vi "Teleop.vi"(10 "Match Info":T1={"Autonomous Elapsed Seconds"=0.0, "TeleOp Elapsed Seconds"=0.0, "Disabled Elapsed Seconds"=0.0, "Visited Autonomous"=FALSE, "Visited TeleOp"=FALSE, "Visited Disabled"=FALSE, "Autonomous Settings"={"Autonomous Style"=enum."Independent", "VI Refnum"=refnum}}, 11 "Call Context":T2) -> ()   [LabVIEW 2013]
doc: "This VI is called for each TeleOp packet received from the DS where the robot is not disabled. It is often used to read from the joysticks and update I/O or to update setpoints for timed control loops. It should complete and return within 20 milliseconds or it may miss DS packets."
uses:
  <vilib>/Rock Robotics/WPI/DriverStation/WPI_DriverStationDerivedRobotMode.ctl
  <vilib>/Rock Robotics/WPI/DriverStation/WPI_DriverStationMatch Info.ctl
  <vilib>/Rock Robotics/WPI/Solenoid/WPI_SolenoidValue.ctl
  Robot Global Data.vi
  <vilib>/Rock Robotics/WPI/Solenoid/WPI_SolenoidSetEnum.vi
  <vilib>/Rock Robotics/WPI/Joystick/WPI_JoystickGetSetRefNum.vi
  <vilib>/Rock Robotics/WPI/Solenoid/WPI_SolenoidGetEnum.vi
  <vilib>/Rock Robotics/WPI/RobotDrive/WPI_RobotDriveGetSetRefNum.vi
  <vilib>/Rock Robotics/WPI/RobotDrive/WPI_RobotDriveMecanumDrive_Cartesian.vi
  <vilib>/Rock Robotics/WPI/RobotDrive/WPI_RobotDriveArcadeDrive_Standard(NoSaturation).vi
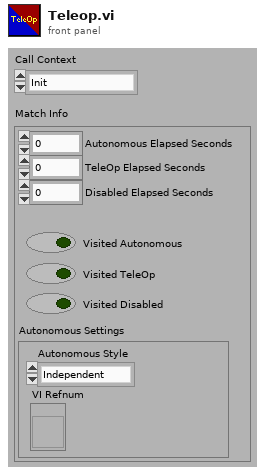
[diagram p1: front panel]
types:
  T1 = typedef "WPI_DriverStationMatch Info.ctl" = cluster{"Autonomous Elapsed Seconds":dbl, "TeleOp Elapsed Seconds":dbl, "Disabled Elapsed Seconds":dbl, "Visited Autonomous":bool, "Visited TeleOp":bool, "Visited Disabled":bool, "Autonomous Settings":cluster{"Autonomous Style":enum16{"Iterative", "Independent"}, "VI Refnum":refnum<vi>}}
  T2 = typedef "WPI_DriverStationDerivedRobotMode.ctl" = enum16{"Init", "Execute", "Stop"}
  T3 = cluster{"axis 1 (x)":dbl, "axis 2 (y)":dbl, "axis 3 (throttle)":dbl, "axis 4":dbl, "axis 5":dbl, "axis 6":dbl}
  T4 = typedef "WPI_JoystickDevRef.ctl" = cluster{"Device":T5}
  T5 = typedef "WPI_JoystickDeviceEnum.ctl" = enum16{"USB 1", "USB 2", "USB 3", "USB 4", "Kinect 1", "Kinect 2"}
  T6 = typedef "WPI_JoystickButtonState.ctl" = cluster{"Button 1":bool, "Button 2":bool, "Button 3":bool, "Button 4":bool, "Button 5":bool, "Button 6":bool, "Button 7":bool, "Button 8":bool, "Button 9":bool, "Button 10":bool, "Button 11":bool, "Button 12":bool}
  T7 = typedef "WPI_RobotDriveDevRef.ctl" = cluster{"DevStatus":errorcluster, "Motors[]":T8[], "Square Inputs":bool, "Max Output":dbl, "Isochronous":bool}
  T8 = typedef "WPI_MotorControlDeviceRef.ctl" = cluster{"DeviceStatus":errorcluster, "Type":enum16{"PWM", "CAN"}, "PWM":cluster{"Digital Module":T9, "PWM Channel":T10, "DeadBand":T11}, "CAN":cluster{"Device Number":u8, "Control Mode":T12, "Semaphore":T13, "Max Vout":dbl}, "Invert":bool, "TransformRef":T14, "InvTransformRef":T14}
  T9 = typedef "FPGA_TypedefDigitalModule.ctl" = enum16{"Digital Module 1", "Digital Module 2"}
  T10 = typedef "FPGA_DIOPWMChannel.ctl" = enum8{"PWM 1", "PWM 2", "PWM 3", "PWM 4", "PWM 5", "PWM 6", "PWM 7", "PWM 8", "PWM 9", "PWM 10", "Invalid"}
  T11 = typedef "WPI_PWMDeadband.ctl" = cluster{"Name":string, "maxPositivePwm":i32, "minPositivePwm":i32, "centerPwm":i32, "maxNegativePwm":i32, "minNegativePwm":i32, "angularRange":u16}
  T12 = typedef "WPI_CANJaguar_ControlMode.ctl" = enum8{"Percent VBus", "Current", "Speed", "Position", "Voltage"}
  T13 = typedef "Semaphore RefNum" = refnum<k1>
  T14 = typedef "WPI_PWMTransform_ConPane.ctl" = refnum<vi>
  T15 = typedef "WPI_SolenoidDevRef.ctl" = cluster{"DevStatus":errorcluster, "Solenoid Module":T16, "Forward Solenoid Channel":T17, "Reverse Solenoid Channel":T17}
  T16 = typedef "FPGA_TypedefSolenoidModule.ctl" = enum16{"Solenoid Module 1", "Solenoid Module 2"}
  T17 = typedef "WPI_SolenoidChannel.ctl" = enum8{"Solenoid 1", "Solenoid 2", "Solenoid 3", "Solenoid 4", "Solenoid 5", "Solenoid 6", "Solenoid 7", "Solenoid 8", "Invalid"}
  T18 = typedef "WPI_SolenoidValue.ctl" = enum16{"Off", "On", "Forward", "Reverse"}
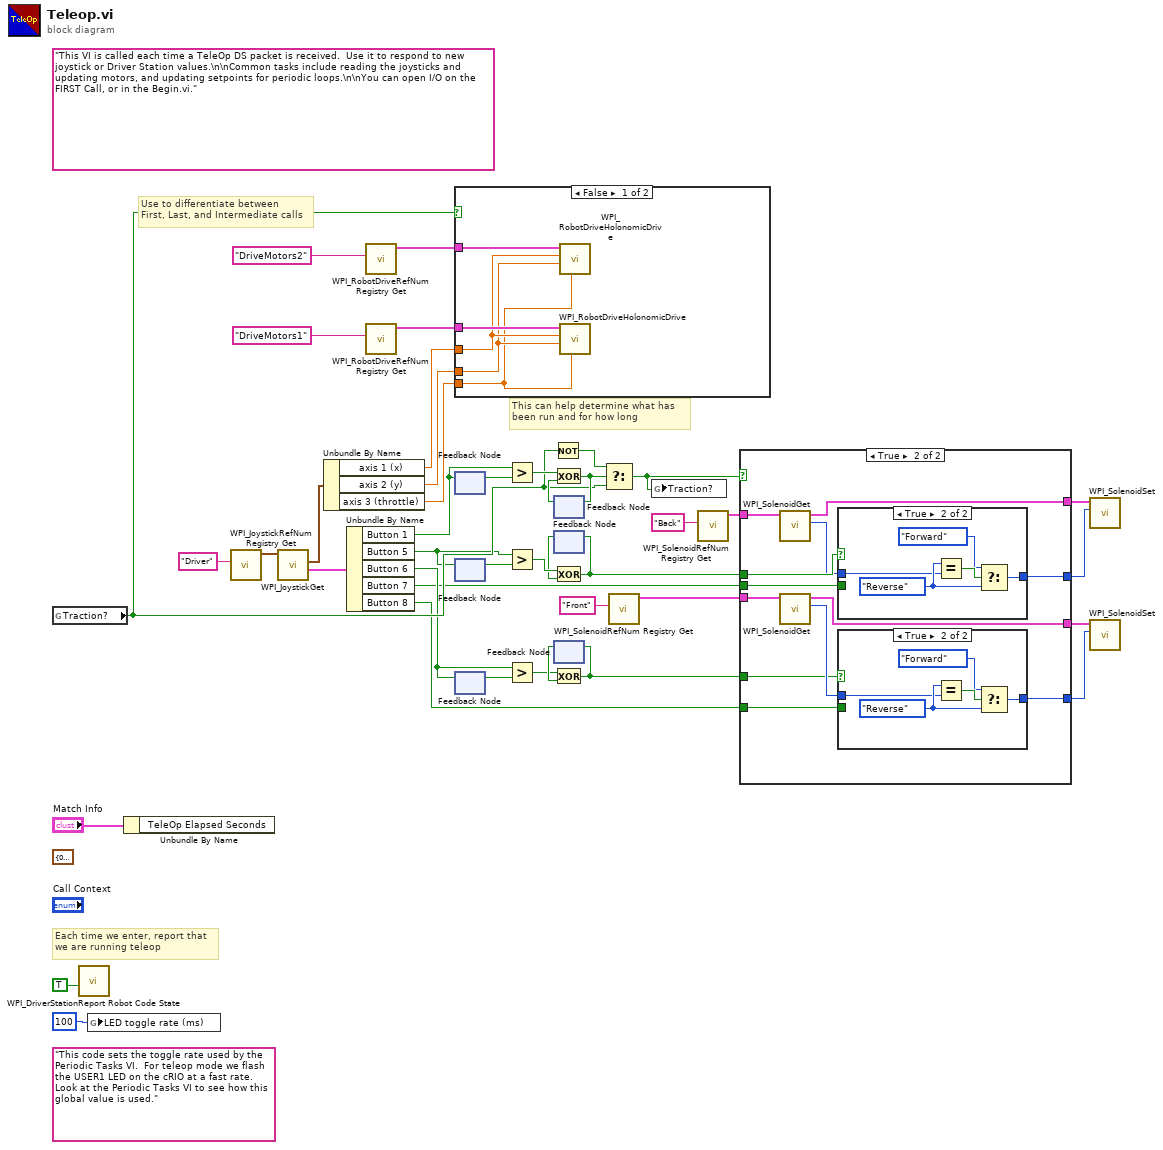
[diagram p0: block diagram]
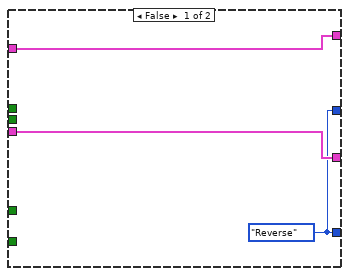
[diagram p2: hidden frame]
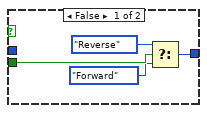
[diagram p3: hidden frame]
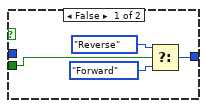
[diagram p4: hidden frame]
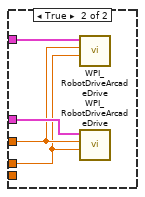
[diagram p5: hidden frame]
diagram:
  (unwired) T3 {"axis 1 (x)"=0.0, "axis 2 (y)"=0.0, "axis 3 (throttle)"=0.0, "axis 4"=0.0, "axis 5"=0.0, "axis 6"=0.0} ("Axes")
  (unwired) "This code sets the toggle rate used by the Periodic Tasks VI.  For teleop mode we flash the USER1 LED on the cRIO at a fast rate.  Look at the Periodic Tasks VI to see how this global value is used."
  (unwired) "This VI is called each time a TeleOp DS packet is received.  Use it to respond to new joystick or Driver Station values.\n\nCommon tasks include reading the joysticks and updating motors, and updating setpoints for periodic loops.\n\nYou can open I/O on the FIRST Call, or in the Begin.vi."
  # "Each time we enter, report that\nwe are running teleop"
  # "Use to differentiate between\nFirst, Last, and Intermediate calls"
  # "This can help determine what has\nbeen run and for how long"
  n1 = global read "Robot Global Data.vi" "Traction?"() -> (w30:bool)
  n2 = call <vilib>:"WPI_DriverStationReport Robot Code State.vi"("TeleOp"=TRUE ("Autonomous")) -> ()  [unwired: 10 in, 1 out]
  n3 = global write "Robot Global Data.vi" "LED toggle rate (ms)"(u32 100 ("LED ms toggle rate")) -> ()
  n4 = Unbundle By Name("Match Info") -> ()  [unwired: 1 out]
  n5 = call <vilib>:"WPI_JoystickRefNum Registry Get.vi"("refnum name"="Driver") -> ("JoystickDevRef"=w40:T4)  [unwired: 1 in, 9 out]
  n6 = call <vilib>:"WPI_JoystickGet.vi"("JoystickDevRef"=w40) -> ("Buttons"=w37:T6, "Axes"=w29:T3)  [unwired: 1 in, 4 out]
  n7 = Unbundle By Name(w29) -> ("axis 1 (x)"=w28:dbl, "axis 2 (y)"=w27:dbl, "axis 3 (throttle)"=w26:dbl)
  n8 = Unbundle By Name(w37) -> ("Button 1"=w31:bool, "Button 5"=w17:bool, "Button 6"=w16:bool, "Button 7"=w4:bool, "Button 8"=w3:bool)
  n9 = call <vilib>:"WPI_RobotDriveRefNum Registry Get.vi"("refnum name"="DriveMotors2") -> ("RobotDriveDevRef"=w1:T7)  [unwired: 1 in, 9 out]
  n10 = call <vilib>:"WPI_RobotDriveRefNum Registry Get.vi"("refnum name"="DriveMotors1") -> ("RobotDriveDevRef"=w24:T7)  [unwired: 1 in, 9 out]
  n11 = case shown="False" w30 {
    tunnel: w28 -> [w45 w49]
    tunnel: w27 -> [w44 w48]
    tunnel: w26 -> [w43 _]
    tunnel: w24 -> [w47 w51]
    tunnel: w1 -> [w46 w50]
    frame False {
      n12 = call-poly <vilib>:"WPI_RobotDriveHolonomicDrive.vi"("Rotation"=w43, "Y"=w44, "X"=w45, "RobotDriveDevRef"=w46) -> ()  [unwired: 5 in, 3 out]
      n13 = call-poly <vilib>:"WPI_RobotDriveHolonomicDrive.vi"("Rotation"=w43, "Y"=w44, "X"=w45, "RobotDriveDevRef"=w47) -> ()  [unwired: 5 in, 3 out]
    }
    frame True {
      n14 = call-poly <vilib>:"WPI_RobotDriveArcadeDrive.vi"("Y axis value"=w48, "X axis value"=w49, "RobotDriveDevRef"=w50) -> ()  [unwired: 6 in, 3 out]
      n15 = call-poly <vilib>:"WPI_RobotDriveArcadeDrive.vi"("Y axis value"=w48, "X axis value"=w49, "RobotDriveDevRef"=w51) -> ()  [unwired: 6 in, 3 out]
    }
  }
  n16 = feedback #1() -> (w32:bool)  [unwired: 1 in]
  n17 = feedback-in #1(w31) -> ()
  n18 = feedback #2() -> (w21:bool)  [unwired: 1 in]
  n19 = feedback-in #2(w17) -> ()
  n20 = feedback #3() -> (w20:bool)  [unwired: 1 in]
  n21 = feedback-in #3(w16) -> ()
  n22 = Greater?(x=w31, y=w32) -> (0:w36:bool)
  n23 = Greater?(x=w17, y=w21) -> (0:w23:bool)
  n24 = Greater?(x=w16, y=w20) -> (0:w18:bool)
  n25 = Not(x=w30) -> (.not. x?=w33:bool)
  n26 = feedback #4() -> (w35:bool)  [unwired: 1 in]
  n27 = Exclusive Or(1:w35, 2:w36) -> (0:w34:bool)
  n28 = feedback-in #4(w34) -> ()
  n29 = feedback #5() -> (w22:bool)  [unwired: 1 in]
  n30 = Exclusive Or(1:w22, 2:w23) -> (0:w6:bool)
  n31 = feedback-in #5(w6) -> ()
  n32 = feedback #6() -> (w19:bool)  [unwired: 1 in]
  n33 = Exclusive Or(1:w19, 2:w18) -> (0:w5:bool)
  n34 = feedback-in #6(w5) -> ()
  n35 = Select(t=w33, s=w34, f=w30) -> (s? t:f=w15:bool)
  n36 = call <vilib>:"WPI_SolenoidRefNum Registry Get.vi"("refnum name"="Front") -> ("SolenoidDevRef"=w11:T15)  [unwired: 9 in, 1 out]
  n37 = global write "Robot Global Data.vi" "Traction?"(w15) -> ()
  n38 = call <vilib>:"WPI_SolenoidRefNum Registry Get.vi"("refnum name"="Back") -> ("SolenoidDevRef"=w12:T15)  [unwired: 9 in, 1 out]
  n39 = case shown="True" w15 {
    tunnel: w12 -> [w54 w66]
    tunnel: w11 -> [w53 w65]
    tunnel: [w54 w64] -> w10
    tunnel: [w53 w63] -> w9
    tunnel: [w52 w60] -> w8
    tunnel: [w52 w56] -> w7
    tunnel: w6 -> [_ w62]
    tunnel: w5 -> [_ w57]
    tunnel: w4 -> [_ w59]
    tunnel: w3 -> [_ w55]
    frame False {
      w52 = WPI_SolenoidValue."Reverse" ("Value")
    }
    frame True {
      n40 = call-poly <vilib>:"WPI_SolenoidGet.vi"("SolenoidDevRef"=w66) -> ("Value"=w61:T18, "SolenoidDevRef"=w64:T15)  [unwired: 8 in, 1 out]
      n41 = call-poly <vilib>:"WPI_SolenoidGet.vi"("SolenoidDevRef"=w65) -> ("Value"=w58:T18, "SolenoidDevRef"=w63:T15)  [unwired: 8 in, 1 out]
      n42 = case shown="True" w62 {
        tunnel: [w78 w81] -> w60
        tunnel: w61 -> [_ w80]
        tunnel: w59 -> [w79 _]
        frame False {
          n43 = Select(t=WPI_SolenoidValue."Reverse" ("Value"), s=w79, f=WPI_SolenoidValue."Forward" ("Value")) -> (s? t:f=w78:T18)
        }
        frame True {
          w82 = WPI_SolenoidValue."Reverse" ("Value")
          n44 = Equal?(x=w82, y=w80) -> (x = y?=w84:bool)
          n45 = Select(t=WPI_SolenoidValue."Forward" ("Value"), s=w84, f=w82) -> (s? t:f=w81:T18)
        }
      }
      n46 = case shown="True" w57 {
        tunnel: [w69 w72] -> w56
        tunnel: w58 -> [_ w71]
        tunnel: w55 -> [w70 _]
        frame False {
          n47 = Select(t=WPI_SolenoidValue."Reverse" ("Value"), s=w70, f=WPI_SolenoidValue."Forward" ("Value")) -> (s? t:f=w69:T18)
        }
        frame True {
          w73 = WPI_SolenoidValue."Reverse" ("Value")
          n48 = Equal?(x=w73, y=w71) -> (x = y?=w75:bool)
          n49 = Select(t=WPI_SolenoidValue."Forward" ("Value"), s=w75, f=w73) -> (s? t:f=w72:T18)
        }
      }
    }
  }
  n50 = call-poly <vilib>:"WPI_SolenoidSet.vi"("Value"=w8, "SolenoidDevRef"=w10) -> ()  [unwired: 8 in, 2 out]
  n51 = call-poly <vilib>:"WPI_SolenoidSet.vi"("Value"=w7, "SolenoidDevRef"=w9) -> ()  [unwired: 8 in, 2 out]
